vi "Set Disabled.vi"(8 "error in (no error)":errorcluster, 10 "Disabled":bool, 11 "NumericIndicator in":refnum<class "NumericIndicator.lvclass">) -> (0 "error out":errorcluster, 3 "NumericIndicator out":refnum<class "NumericIndicator.lvclass">)   [LabVIEW 2020, in "VolatusGUIElements.lvlib" / "NumericIndicator.lvclass"]
uses:
  NumericIndicator.lvclass
  NumericIndicator.lvclass/NumericIndicator.ctl
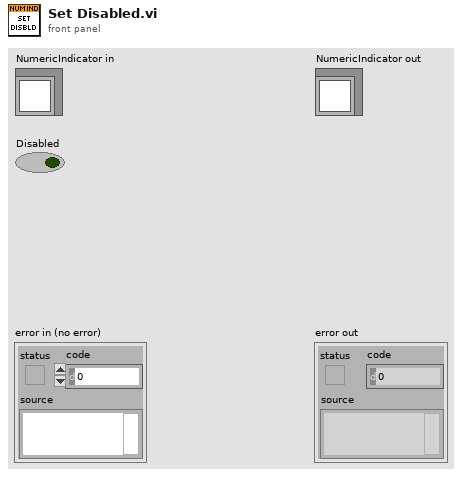
[diagram p1: front panel]
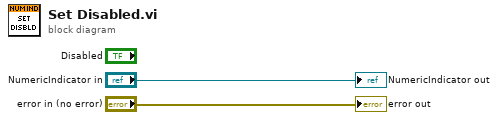
[diagram p0: block diagram]
diagram:
  "error out" <- "error in (no error)"
  "NumericIndicator out" <- "NumericIndicator in"
